vi "Update Window Title.vi"(8 "error in (no error)":errorcluster, 9 "Experiment Name":string, 10 "Experiment File Path":path, 11 "VI in":refnum<vi>) -> (0 "error out":errorcluster)   [LabVIEW 2020, in "RxnRover.lvlib"]
doc: "Updates the window title with the correct experiment name and path."
uses:
  RxnRover.lvlib
  logging/logging.lvlib
panel:
  out "Title String":string
  # "Debug"
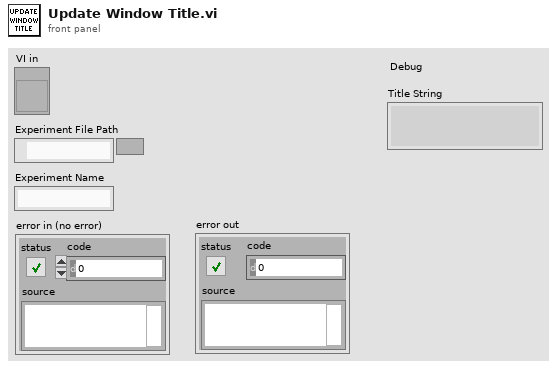
[diagram p1: front panel]
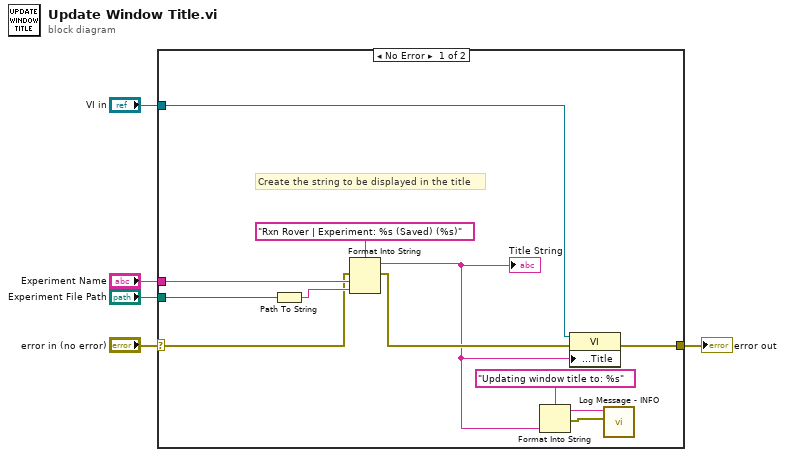
[diagram p0: block diagram]
diagram:
  n1 = case shown="No Error" "error in (no error)" {
    selector: "error in (no error)" -> [w10 w18]
    tunnel: "Experiment File Path" -> [w17 _]
    tunnel: "VI in" -> [w16 _]
    tunnel: [w15 w18] -> w3
    tunnel: "Experiment Name" -> [w13 _]
    frame No Error {
      # "Create the string to be displayed in the title"
      n2 = Path To String(path=w17) -> (string=w12:string)
      n3 = Format Into String(format string="Rxn Rover | Experiment: %s (Saved) (%s)", error in=w10, w13, w12) -> (resulting string=w6:string, error out=w11:errorcluster)  [unwired: 1 in]
      "Title String" <- w6
      n4 = Format Into String(format string="Updating window title to: %s", w6) -> (resulting string=w8:string, error out=w7:errorcluster)  [unwired: 2 in]
      n5 = property class="VI"(reference=w16, error in=w11, "Front Panel.Title"=w6) -> (error out=w15:errorcluster)  [unwired: 1 out]
      n6 = call "Log Message - INFO.vi"("error in (no error)"=w7, "Message"=w8) -> ()  [unwired: 9 in, 1 out]
    }
    frame Error {
    }
  }
  "error out" <- w3
